vi "Acceleration_All_Pulse_Boyer_Mods2.vi"() -> ()   [LabVIEW 2015]
uses:
  Control 1 Trigger Source.ctl
  <vilib>/DAQmx/read.llb/DAQmx Read (Analog 1D Wfm NChan NSamp).vi
  <vilib>/DAQmx/create/channels.llb/DAQmx Create Channel (AI-Voltage-Basic).vi
  <vilib>/DAQmx/configure/timing.llb/DAQmx Timing (Sample Clock).vi
  <vilib>/DAQmx/miscellaneous.llb/DAQmx Fill In Error Info.vi
  <vilib>/Waveform/WDTOps.llb/WDT Append Waveforms DBL.vi
  <vilib>/measure/mascope.llb/Pulse Measurements 1 chan.vi
  <vilib>/measure/NI_MAPro.lvlib
panel:
  in  "# of Periods/Avg":dbl
  in  "Pulse/Rev":dbl=25.0
  out "Waveform":waveform(dbl)(graph)
  out "Speed":dbl[](array[numeric])
  out "Period":dbl[](array[numeric])
  out "Boolean":bool
  in  "Tab Control":enum32{"Page 1", "Page 2", "Page 3"}(tab)
  out "Waveform Graph":waveform(dbl)(graph)
  out "Waveform Graph 2":waveform(dbl)(graph)
  out "Waveform Chart 2":dbl(graph)
  out "Waveform Chart":dbl(graph)
  out "data":waveform(dbl)
  out "RPM 2":dbl format="%.2f"
  in  "stop":bool
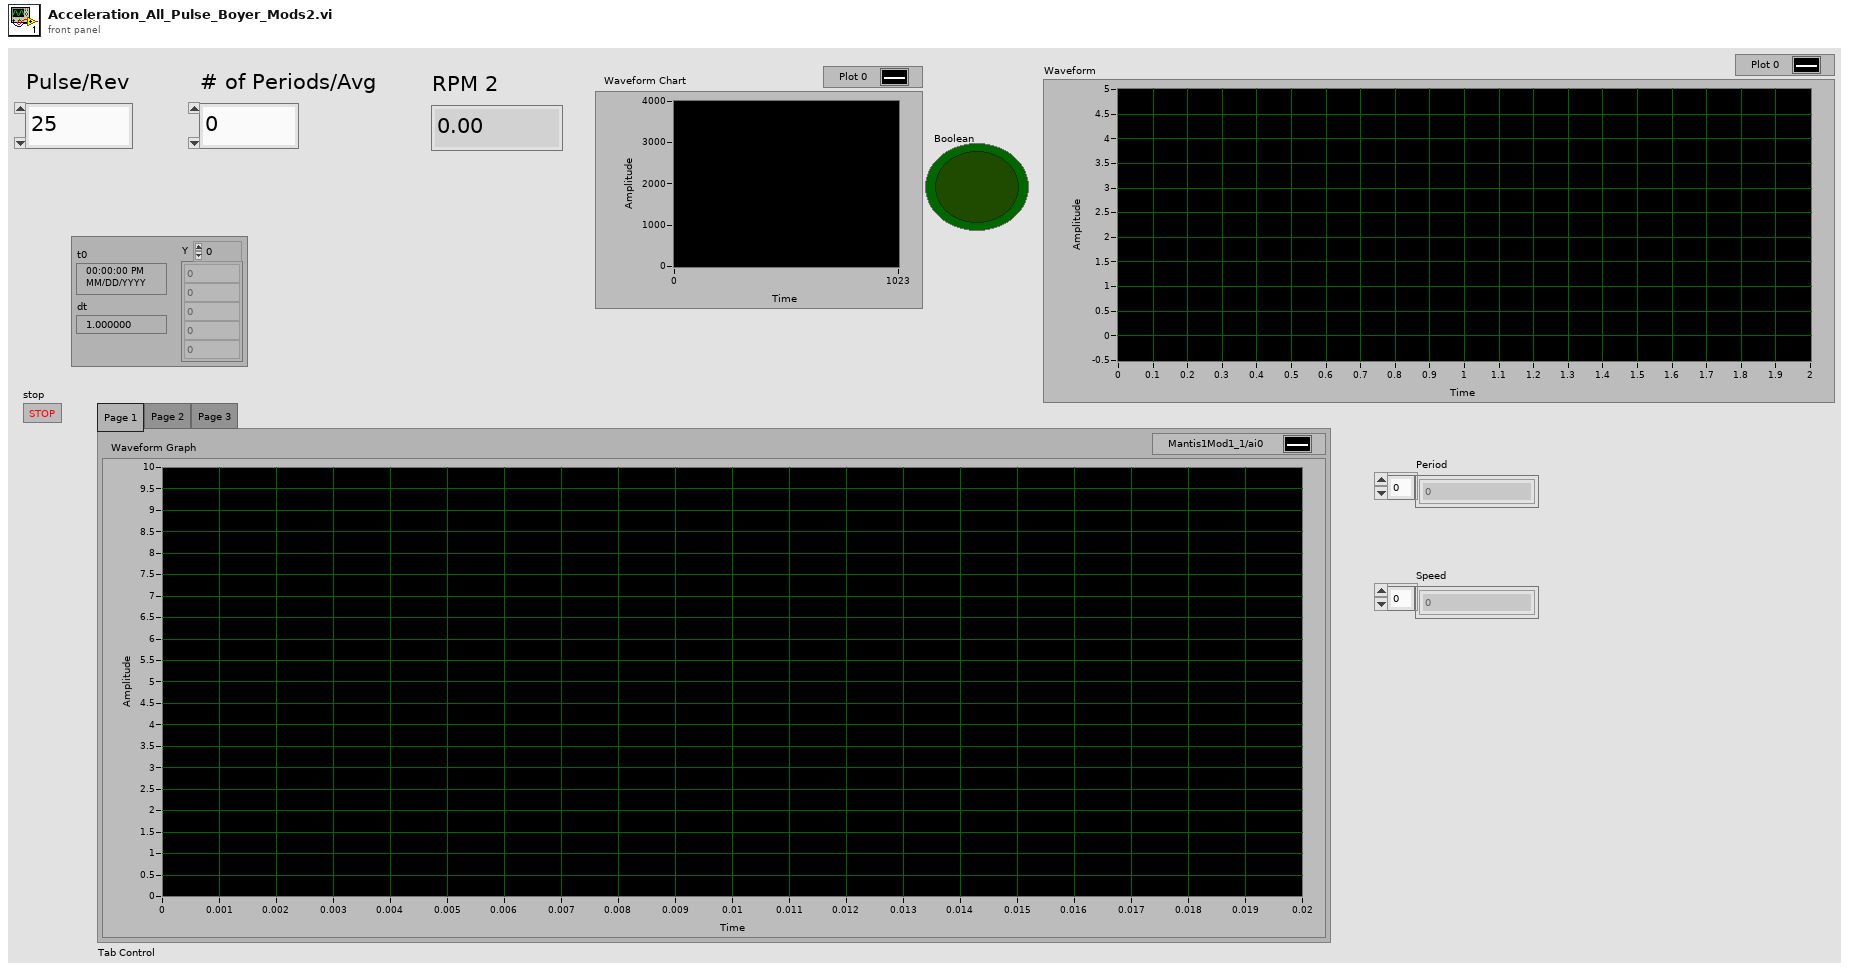
[diagram p1: front panel]
types:
  T1 = typedef "Control 1 Trigger Source.ctl" = cluster{"E-Stop":waveform(dbl), "Stop":waveform(dbl)}
  T2 = cluster{"high ref level":dbl, "mid ref level":dbl, "low ref level":dbl, "ref units":u16}
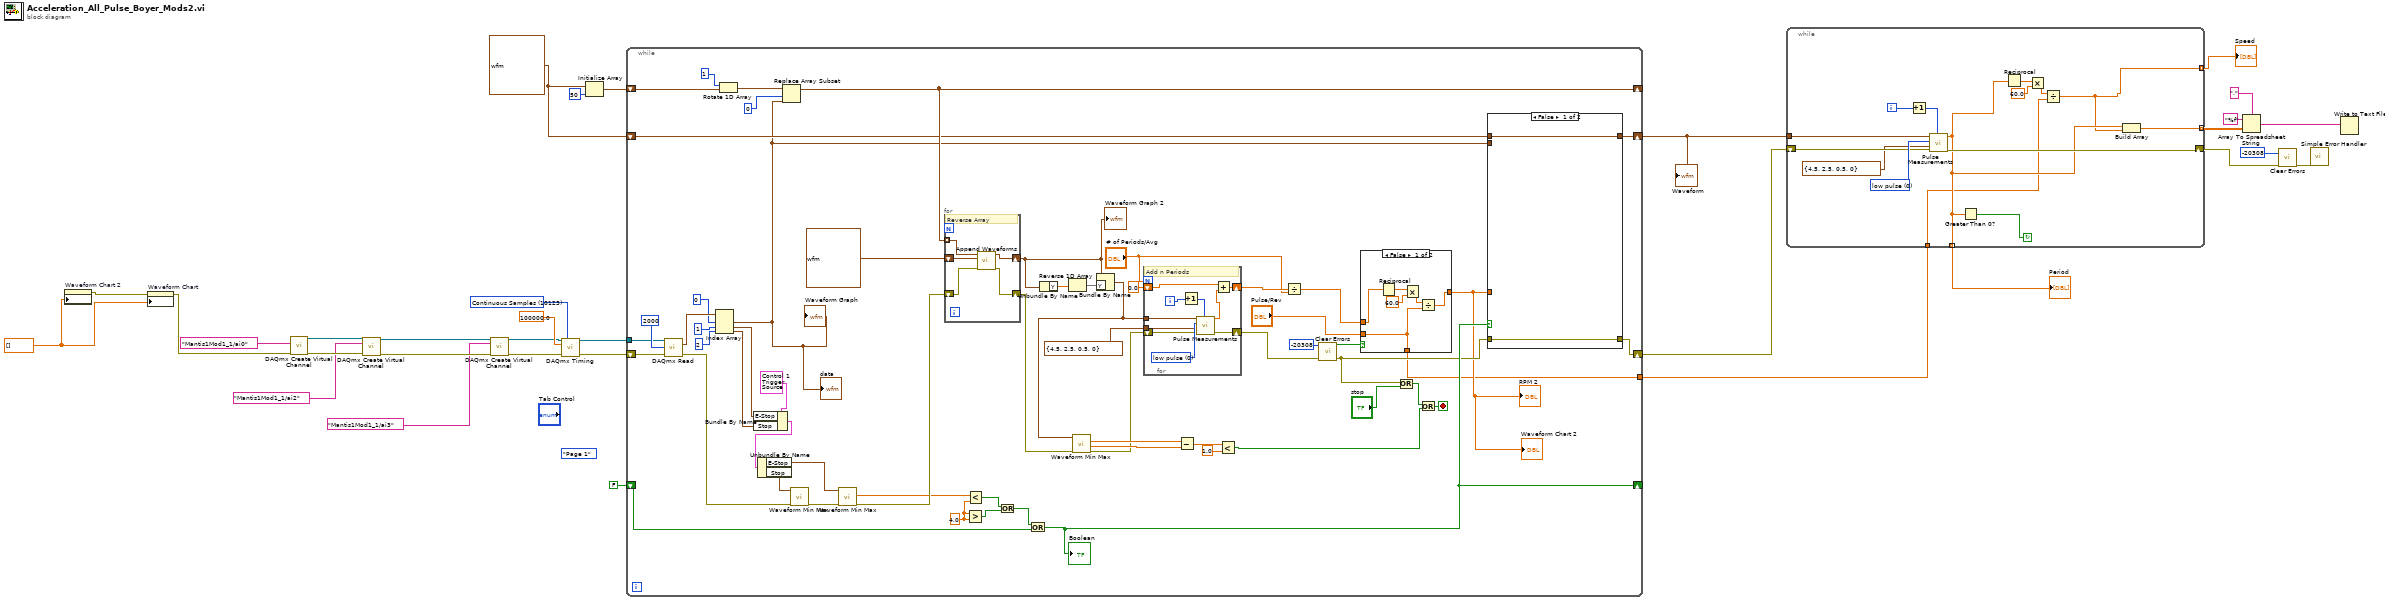
[diagram p0: block diagram]
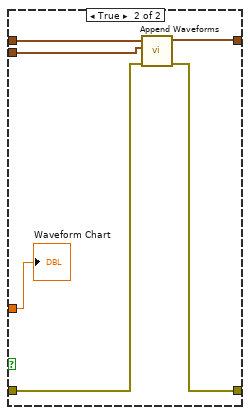
[diagram p2: hidden frame]
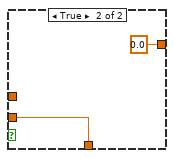
[diagram p3: hidden frame]
diagram:
  (unwired) enum32{"Page 1", "Page 2", "Page 3"}."Page 1" ("Tab Control")
  w5 = dbl[] [] ("History Data")
  w16 = waveform(dbl) {"t0"=timestamp(0 s since 1904-01-01), "dt"=1e-05, "Y"=[]} ("Waveform")
  w30 = 10123 items=["Finite Samples"=10178, "Continuous Samples"=10123, "Hardware Timed Single Point"=12522] ("sample mode")
  n1 = property on="Waveform Chart 2" class="WFChart (strict)"("History Data"=w5) -> (error out=w6:errorcluster)  [unwired: 2 in, 1 out]
  n2 = property on="Waveform Chart" class="WFChart (strict)"(error in=w6, "History Data"=w5) -> (error out=w13:errorcluster)  [unwired: 1 in, 1 out]
  n3 = call-poly <vilib>:"DAQmx Create Virtual Channel.vi"("physical channels"=tag "Mantis1Mod1_1/ai0", "error in"=w13) -> ("task out"=w25:refnum<k21>, "error out"=w24:errorcluster)  [unwired: 12 in]
  n4 = call-poly <vilib>:"DAQmx Create Virtual Channel.vi"("task in"=w25, "physical channels"=tag "Mantis1Mod1_1/ai2", "error in"=w24) -> ("task out"=w22:refnum<k21>, "error out"=w21:errorcluster)  [unwired: 11 in]
  n5 = call-poly <vilib>:"DAQmx Create Virtual Channel.vi"("task in"=w22, "physical channels"=tag "Mantis1Mod1_1/ai3", "error in"=w21) -> ("task out"=w19:refnum<k21>, "error out"=w20:errorcluster)  [unwired: 11 in]
  n6 = call-poly <vilib>:"DAQmx Timing.vi"("task/channels in"=w19, "sample mode"=w30, "rate"=100000.0, "error in"=w20) -> ("task out"=w29:refnum<k21>, "error out"=w28:errorcluster)  [unwired: 10 in]
  n7 = Initialize Array(w16, 50 ("dimension size")) -> (w26:waveform(dbl)[])
  n8 = while {
    tunnel: w29 -> [w90]
    shift-right: [w84] -> _
    shift-left: w26 -> [w88]
    shift-right: [w43] -> w15
    shift-left: w28 -> [w89]
    shift-right: [w70] -> _
    shift-left: FALSE -> [w74]
    shift-right: [w42] -> w14
    shift-left: w16 -> [w41]
    tunnel: [w37] -> w4
    stop <- w52 stop-if-true
    w33 = 4.0 ("y")
    n9 = call-poly <vilib>:"DAQmx Read.vi"("task/channels in"=w90, "number of samples per channel"=2000, "error in"=w89) -> ("data"=w78:waveform(dbl)[], "error out"=w75:errorcluster)  [unwired: 10 in, 1 out]
    n10 = Index Array(array=w78, index #1=0 ("index"), index #2=1 ("index"), index #3=2 ("index")) -> (element #1=w40:waveform(dbl), element #2=w65:waveform(dbl), element #3=w64:waveform(dbl))
    "Waveform Graph" <- w40
    "data" <- w40
    n11 = Rotate 1D Array(1:w88, 2:1 ("n")) -> (0:w86:waveform(dbl)[])
    n12 = Bundle By Name(cluster=T1 {"E-Stop"={"t0"=timestamp(0 s since 1904-01-01), "dt"=1.0, "Y"=[]}, "Stop"={"t0"=timestamp(0 s since 1904-01-01), "dt"=1.0, "Y"=[]}}, "E-Stop"=w65, "Stop"=w64) -> (w59:T1)
    n13 = Unbundle By Name(w59) -> ("E-Stop"=w61:waveform(dbl), "Stop"=w62:waveform(dbl))
    n14 = Replace Array Subset(array=w86, new element=w40, index=0) -> (w84:waveform(dbl)[])
    n15 = call <vilib>:"Waveform Min Max.vi"("error in (no error)"=w75, "waveform in"=w62) -> ("error out"=w63:errorcluster)  [unwired: 4 in, 5 out]
    n16 = call <vilib>:"Waveform Min Max.vi"("error in (no error)"=w63, "waveform in"=w61) -> ("error out"=w48:errorcluster, "Y max"=w34:dbl)  [unwired: 4 in, 4 out]
    n17 = for {
      tunnel: w84 -> [w120] mode=indexing
      shift-right: [w119] -> w47
      shift-left: w48 -> [w121]
      shift-right: [w118] -> w45
      shift-left: waveform(dbl) {"t0"=timestamp(0 s since 1904-01-01), "dt"=1e-05, "Y"=[]} ("Waveform") -> [w122]
      # "Reverse Array"
      n18 = call-poly <vilib>:"Append Waveforms.vi"("error in (no error)"=w121, "waveform B"=w122, "waveform A"=w120) -> ("error out"=w119:errorcluster, "waveform out"=w118:waveform(dbl))  [unwired: 7 in]
    }
    "Waveform Graph 2" <- w45
    n19 = Greater?(x=w33, y=w33) -> (0:w57:bool)
    n20 = Less?(x=w34, y=w33) -> (x < y?=w58:bool)
    n21 = Or(x=w58, y=w57) -> (x .or. y?=w56:bool)
    n22 = Or(x=w56, y=w74) -> (x .or. y?=w70:bool)
    "Boolean" <- w70
    n23 = Unbundle By Name(w45) -> ("Y"=w72:dbl[])
    n24 = Reverse 1D Array(array=w72) -> (reversed array=w71:dbl[])
    n25 = Bundle By Name(cluster=w45, "Y"=w71) -> (w39:waveform(dbl))
    n26 = call <vilib>:"Waveform Min Max.vi"("error in (no error)"=w47, "waveform in"=w39) -> ("error out"=w46:errorcluster, "Y min"=w54:dbl, "Y max"=w55:dbl)  [unwired: 4 in, 3 out]
    n27 = for {
      N: "# of Periods/Avg" -> [_]
      tunnel: T2 {"high ref level"=4.5, "mid ref level"=2.5, "low ref level"=0.5, "ref units"=0} ("reference levels") -> [w99]
      tunnel: w39 -> [w97]
      shift-right: [w100] -> w83
      shift-left: w46 -> [w98]
      shift-right: [w94] -> w68
      shift-left: 0.0 ("period") -> [w93]
      i -> [w96]
      w101 = u16 0 items=["low pulse", "high pulse"] ("polarity (high)")
      # "Add n Periods"
      n28 = Increment(x=w96) -> (x+1=w95:i32)
      n29 = call-poly <vilib>:"Pulse Measurements.vi"("pulse number (1)"=w95, "error in (no error)"=w98, "reference levels"=w99, "polarity (high)"=w101, "signal in"=w97) -> ("error out"=w100:errorcluster, "period"=w92:dbl)  [unwired: 2 in, 3 out]
      n30 = Add(x=w93, y=w92) -> (x+y=w94:dbl)
    }
    n31 = Subtract(x=w55, y=w54) -> (x-y=w51:dbl)
    n32 = Less?(x=w51, y=1.0) -> (x < y?=w49:bool)
    n33 = Divide(x=w68, y="# of Periods/Avg") -> (x/y=w67:dbl)
    n34 = call <vilib>:"Clear Errors.vi"("error in (no error)"=w83, "specific error code to clear (0: all)"=-20308) -> ("error out"=w44:errorcluster, "specific error cleared?"=w81:bool)  [unwired: 4 in]
    n35 = case shown="False" w81 {
      tunnel: w67 -> [w115 _]
      tunnel: [w112 0.0] -> w38
      tunnel: [w110 w116] -> w37
      tunnel: "Pulse/Rev" -> [w110 w116]
      frame False {
        n36 = Reciprocal(x=w115) -> (1/x=w113:dbl)
        n37 = Multiply(x=w113, y=60.0) -> (x*y=w111:dbl)
        n38 = Divide(x=w111, y=w110) -> (x/y=w112:dbl)
      }
      frame True {
      }
    }
    "RPM 2" <- w38
    "Waveform Chart 2" <- w38
    n39 = Or(x=w44, y="stop") -> (x .or. y?=w53:bool)
    n40 = Or(x=w53, y=w49) -> (x .or. y?=w52:bool)
    n41 = case shown="False" w70 {
      tunnel: w38 -> [_ w109]
      tunnel: w44 -> [w103 w106]
      tunnel: [w103 w105] -> w43
      tunnel: [w102 w107] -> w42
      tunnel: w41 -> [w102 w108]
      tunnel: w40 -> [_ w104]
      frame False {
      }
      frame True {
        n42 = call-poly <vilib>:"Append Waveforms.vi"("error in (no error)"=w106, "waveform B"=w104, "waveform A"=w108) -> ("error out"=w105:errorcluster, "waveform out"=w107:waveform(dbl))  [unwired: 7 in]
        "Waveform Chart" <- w109
      }
    }
  }
  "Waveform" <- w14
  n43 = while {
    tunnel: w14 -> [w136]
    shift-right: [w131] -> w3
    shift-left: w15 -> [w135]
    tunnel: [w126] -> w12 mode=indexing
    tunnel: [w125] -> w11 mode=indexing
    tunnel: [w124] -> w9 mode=indexing
    tunnel: w4 -> [w123]
    i -> [w133]
    stop <- w130 continue-if-true
    w137 = u16 0 items=["low pulse", "high pulse"] ("polarity (high)")
    n44 = Increment(x=w133) -> (x+1=w132:i32)
    n45 = call-poly <vilib>:"Pulse Measurements.vi"("pulse number (1)"=w132, "error in (no error)"=w135, "reference levels"=T2 {"high ref level"=4.5, "mid ref level"=2.5, "low ref level"=0.5, "ref units"=0}, "polarity (high)"=w137, "signal in"=w136) -> ("error out"=w131:errorcluster, "period"=w126:dbl)  [unwired: 2 in, 3 out]
    n46 = Greater Than 0?(x=w126) -> (x > 0?=w130:bool)
    n47 = Reciprocal(x=w126) -> (1/x=w128:dbl)
    n48 = Multiply(x=w128, y=60.0) -> (x*y=w127:dbl)
    n49 = Divide(x=w127, y=w123) -> (x/y=w125:dbl)
    n50 = Build Array(w126, w125) -> (w124:dbl[])
  }
  "Period" <- w12
  "Speed" <- w11
  n51 = Array To Spreadsheet String(delimiter (Tab)=",", array=w9, 3:"%f" ("format string")) -> (spreadsheet string=w8:string)
  n52 = call <vilib>:"Clear Errors.vi"("error in (no error)"=w3, "specific error code to clear (0: all)"=-20308) -> ("error out"=w1:errorcluster)  [unwired: 4 in, 1 out]
  n53 = call <vilib>:"Simple Error Handler.vi"("error in (no error)"=w1) -> ()  [unwired: 4 in, 5 out]
  n54 = Write to Text File(text=w8) -> ()  [unwired: 3 in, 3 out]
